vi "SortZtoATest.vi"(11 "error in":errorcluster) -> (15 "error out":errorcluster)   [LabVIEW 2023, in "TestVIs.lvlib"]
uses:
  <vilib>/addons/_JKI Toolkits/Caraya/classes/Assert/Assert Equal Value_Variant.vi
  TestVIs.lvlib
  <vilib>/addons/_JKI Toolkits/Caraya/classes/Test/Test.lvclass
  <vilib>/addons/_JKI Toolkits/Caraya/classes/Assert/Assert.lvclass
  Library/Unit Testing CA1.lvlib
panel:
  # "REVERSE SORT TEST"
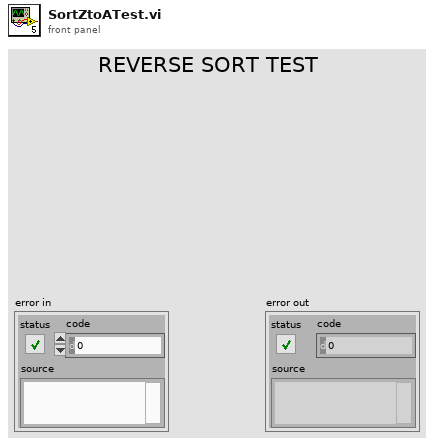
[diagram p1: front panel]
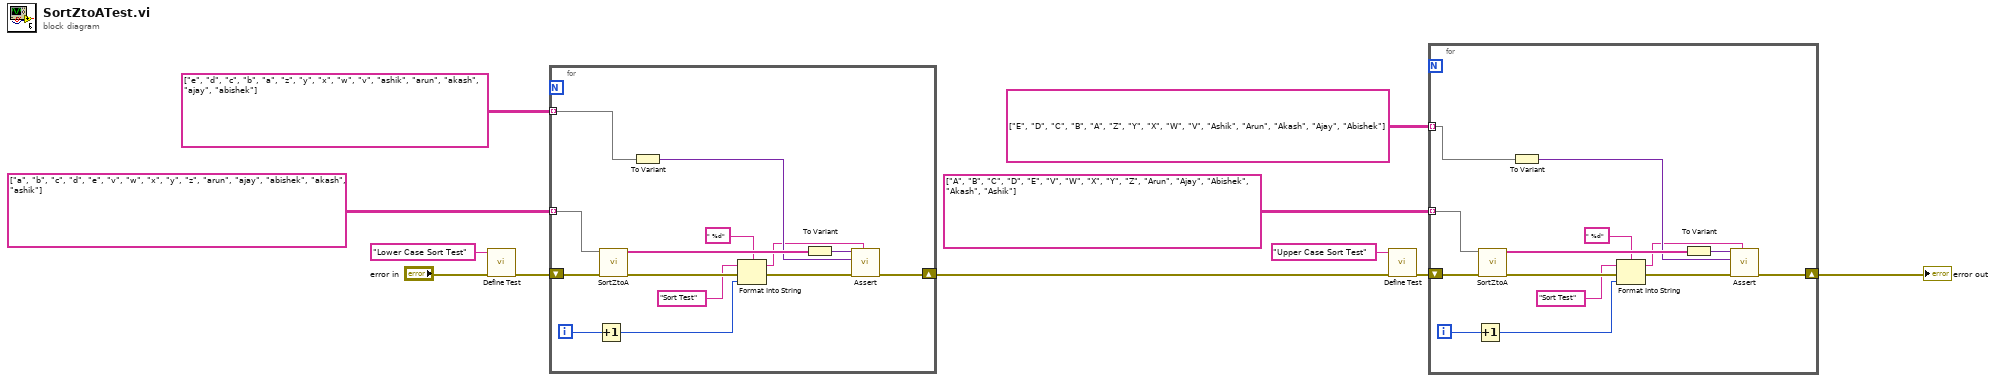
[diagram p0: block diagram]
diagram:
  n1 = call <vilib>:"Define Test.vi"("error in (no error)"="error in", "Label (VI Title)"="Lower Case Sort Test") -> ("error out"=w9:errorcluster)  [unwired: 8 in, 1 out]
  n2 = for {
    shift-right: [w13] -> w2
    shift-left: w9 -> [w25]
    tunnel: string[][] [["a", "b", "c", "d", "e"], ["v", "w", "x", "y", "z"], ["arun", "ajay", "abishek", "akash", "ashik"]] ("Input Array") -> [w12] mode=indexing
    tunnel: string[][] [["e", "d", "c", "b", "a"], ["z", "y", "x", "w", "v"], ["ashik", "arun", "akash", "ajay", "abishek"]] ("Input Array") -> [w14] mode=indexing
    i -> [w18]
    n3 = Increment(x=w18) -> (x+1=w15:i32)
    n4 = call "SortZtoA.vi"("Input Array"=w12, "error in"=w25) -> ("reversed array"=w24:string[], "error out"=w21:errorcluster)  [unwired: 12 in]
    n5 = To Variant(anything=w14) -> (Variant=w23:variant)
    n6 = Format Into String(format string=" %d", initial string="Sort Test" ("Label"), error in=w21, w15) -> (resulting string=w16:string, error out=w20:errorcluster)
    n7 = To Variant(anything=w24) -> (Variant=w22:variant)
    n8 = call-poly <vilib>:"Assert.vi"("Label"=w16, "error in (no error)"=w20, "Y"=w23, "X"=w22) -> ("error out"=w13:errorcluster)  [unwired: 6 in, 1 out]
  }
  n9 = call <vilib>:"Define Test.vi"("error in (no error)"=w2, "Label (VI Title)"="Upper Case Sort Test") -> ("error out"=w5:errorcluster)  [unwired: 8 in, 1 out]
  n10 = for {
    shift-right: [w27] -> w1
    shift-left: w5 -> [w39]
    tunnel: string[][] [["A", "B", "C", "D", "E"], ["V", "W", "X", "Y", "Z"], ["Arun", "Ajay", "Abishek", "Akash", "Ashik"]] ("Input Array") -> [w26] mode=indexing
    tunnel: string[][] [["E", "D", "C", "B", "A"], ["Z", "Y", "X", "W", "V"], ["Ashik", "Arun", "Akash", "Ajay", "Abishek"]] ("Input Array") -> [w28] mode=indexing
    i -> [w32]
    n11 = Increment(x=w32) -> (x+1=w29:i32)
    n12 = call "SortZtoA.vi"("Input Array"=w26, "error in"=w39) -> ("reversed array"=w38:string[], "error out"=w35:errorcluster)  [unwired: 12 in]
    n13 = To Variant(anything=w28) -> (Variant=w37:variant)
    n14 = Format Into String(format string=" %d", initial string="Sort Test" ("Label"), error in=w35, w29) -> (resulting string=w30:string, error out=w34:errorcluster)
    n15 = To Variant(anything=w38) -> (Variant=w36:variant)
    n16 = call-poly <vilib>:"Assert.vi"("Label"=w30, "error in (no error)"=w34, "Y"=w37, "X"=w36) -> ("error out"=w27:errorcluster)  [unwired: 6 in, 1 out]
  }
  "error out" <- w1
